vi "Config.File.Write.vi"(8 "error in":errorcluster, 11 "path":path) -> (0 "error out":errorcluster)   [LabVIEW 2016]
uses:
  Tma.lib/nlconfig.llb/fp2ini mode.ctl
  Config.Global.vi
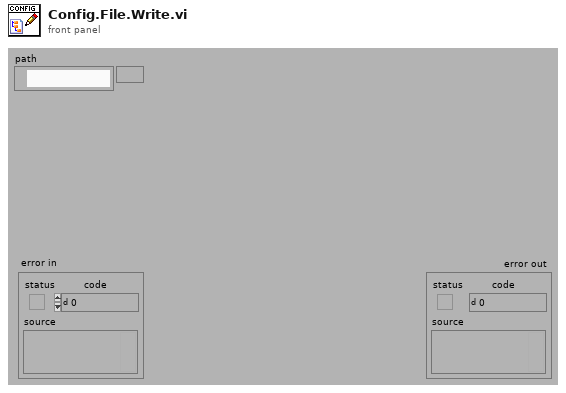
[diagram p1: front panel]
types:
  T1 = typedef "fp2ini mode.ctl" = enum16{"Read Controls", "Write Controls", "Write Indicators", "Read Indicators", "Write all", "Read all"}
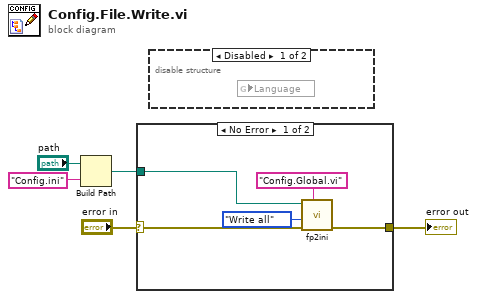
[diagram p0: block diagram]
diagram:
  n1 = Build Path(base path="path", name or relative path="Config.ini") -> (appended path=w1:path)
  n2 = case shown="No Error" "error in" {
    selector: "error in" -> [w8 w11]
    tunnel: [w7 w11] -> w5
    tunnel: w1 -> [w6 _]
    frame No Error {
      n3 = call "fp2ini.vi"("vi-name (caller if empty)"="Config.Global.vi", "error in"=w8, "mode"=fp2ini_mode."Write all", "ini-file path"=w6) -> ("error out"=w7:errorcluster)  [unwired: 7 in]
    }
    frame Error {
    }
  }
  "error out" <- w5
  n4 = disable-structure shown="Disabled" {
    frame Disabled {
      n5 = global read "Config.Global.vi" "Language"() -> ()  [unwired: 1 in]
    }
    frame Enabled {
    }
  }
